vi "Log_file_player.vi"() -> ()   [LabVIEW 2013]
uses:
  ctl/log_data.ctl
panel:
  out "웨이브폼 그래프":waveform(dbl)(graph)
  out "웨이브폼 차트":waveform(dbl)(graph)
  out "에러 출력":errorcluster
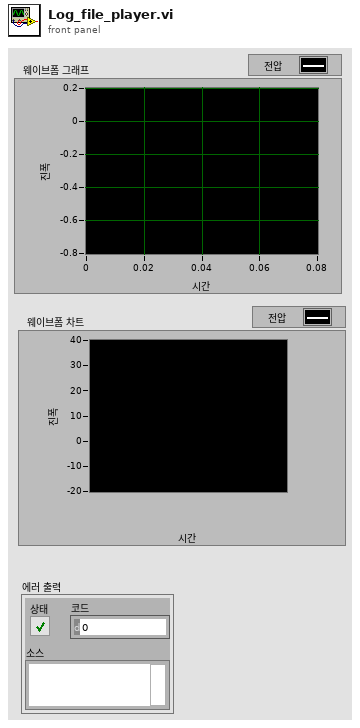
[diagram p1: front panel]
types:
  T1 = typedef "log_data.ctl" = cluster{"strain filter_n_nulling wf":waveform(dbl)[], "force wf":waveform(dbl), "force":dbl, "Balance xy wfs":cluster{"X":dbl, "Y":dbl}[], "vacuum kpa wf":waveform(dbl), "pcb temp":dbl[][]}
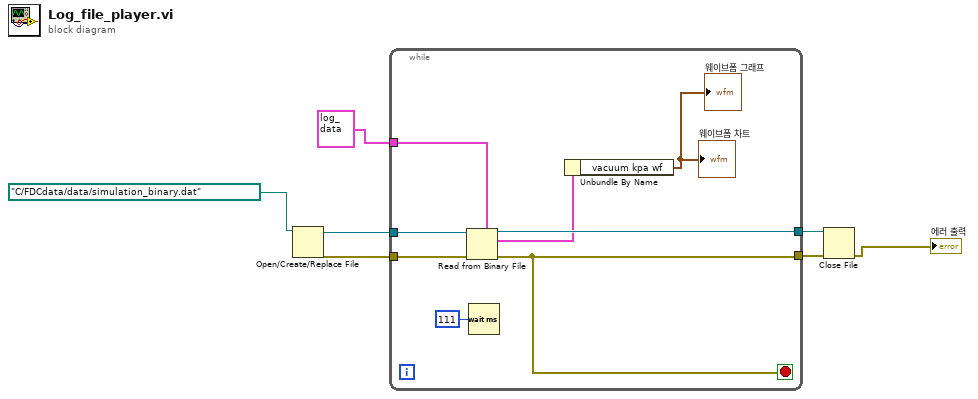
[diagram p0: block diagram]
diagram:
  n1 = Open/Create/Replace File(file path (use dialog)=path "C:/FDCdata/data/simulation_binary.dat" ("파일 경로(대화 상자 사용)")) -> (refnum out=w7:refnum<file>, error out=w6:errorcluster)  [unwired: 5 in, 1 out]
  n2 = while {
    tunnel: w7 -> [w15]
    tunnel: w6 -> [w14]
    tunnel: T1 {"strain filter_n_nulling wf"=[{"t0"=timestamp(0 s since 1904-01-01), "dt"=1.0, "Y"=[0.0, 0.0, 0.0, 6.0]}], "force wf"={"t0"=timestamp(0 s since 1904-01-01), "dt"=1.0, "Y"=[0.0, 0.0, 0.0, 5.0]}, "force"=2.0, "Balance xy wfs"=[{"X"=2.0, "Y"=0.0}], "vacuum kpa wf"={"t0"=timestamp(0 s since 1904-01-01), "dt"=1.0, "Y"=[0.0, 0.0, 0.0, 3.0]}, "pcb temp"=[]} ("log data") -> [w13]
    tunnel: [w10] -> w4
    tunnel: [w12] -> w3
    stop <- w10 stop-if-true
    n3 = Read from Binary File(5:w13, 8:w14, 11:w15) -> (0:w10:errorcluster, 2:w9:T1, 3:w12:refnum<file>)  [unwired: 3 in, 1 out]
    n4 = Wait (ms)(milliseconds to wait=u32 111 ("대기 시간(ms)")) -> ()  [unwired: 1 out]
    n5 = Unbundle By Name(w9) -> ("vacuum kpa wf"=→"웨이브폼 차트" →"웨이브폼 그래프":waveform(dbl))
  }
  n6 = Close File(refnum=w3, error in=w4) -> (error out=→"에러 출력":errorcluster)  [unwired: 1 out]
